vi "SSH Get Pipe Descriptor.vi"(8 "Error In":errorcluster, 11 "SSH Session":refnum<k1>) -> (0 "Error Out":errorcluster, 2 "SSH Pipe Descriptor":i32=-1, 3 "SSH Session":refnum<k1>)   [LabVIEW 2020, in "LMH-LINX.lvlib"]
uses:
  LMH-LINX.lvlib
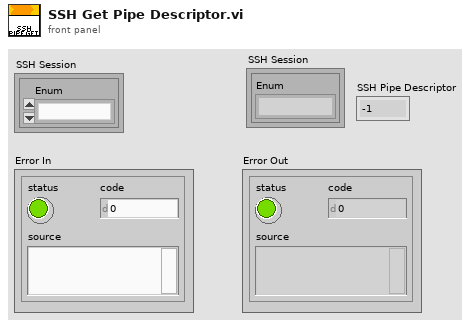
[diagram p1: front panel]
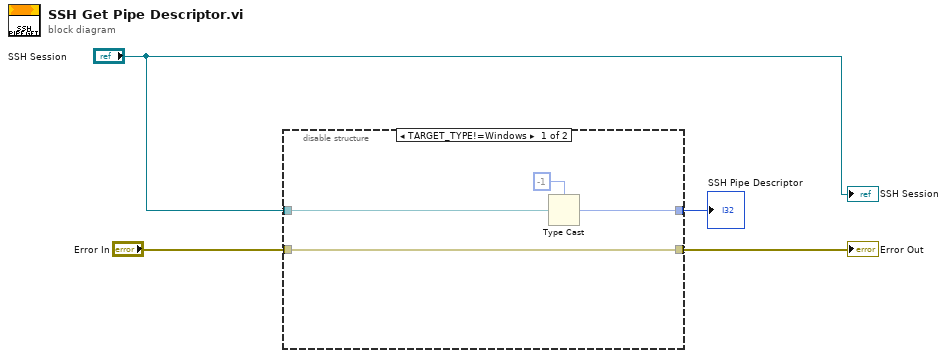
[diagram p0: block diagram]
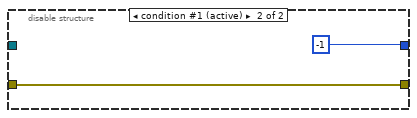
[diagram p2: hidden frame]
diagram:
  n1 = disable-structure shown="TARGET_TYPE!=Windows" {
    disable-tunnel: [w7 w10] -> w3
    disable-tunnel: "Error In" -> [w7 w10]
    disable-tunnel: "SSH Session" -> [w8 _]
    disable-tunnel: [w6 -1 ("SSH Pipe Descriptor")] -> w2
    frame condition #0 {
      n2 = Type Cast(type=-1 ("SSH Pipe Descriptor"), x=w8) -> (*(type *) &x=w6:i32)
    }
    frame condition #1 (active) {
    }
  }
  "Error Out" <- w3
  "SSH Pipe Descriptor" <- w2
  "SSH Session" <- "SSH Session"
